vi "MISSION_ITEM Jump.vi"(0 "Waypoint to jump to":sgl, 5 "Number of times to repeat":sgl) -> (4 "Mission Item":T1={"target_system"=0, "target_component"=0, "sequence"=0, "frame"=enum."GLOBAL RELATIVE ALT", "command"=0, "current"=FALSE, "autocontinue"=FALSE, "param1"=0.0, "param2"=0.0, "param3"=0.0, "param4"=0.0, "Lat"=0.0, "Lon"=0.0, "Altitude (m)"=0.0})   [LabVIEW 2014]
uses:
  Controls/Mission Planning Controls/MAVLINK Mission Item.ctl
  Controls/MAVLINK Mav Frame.ctl
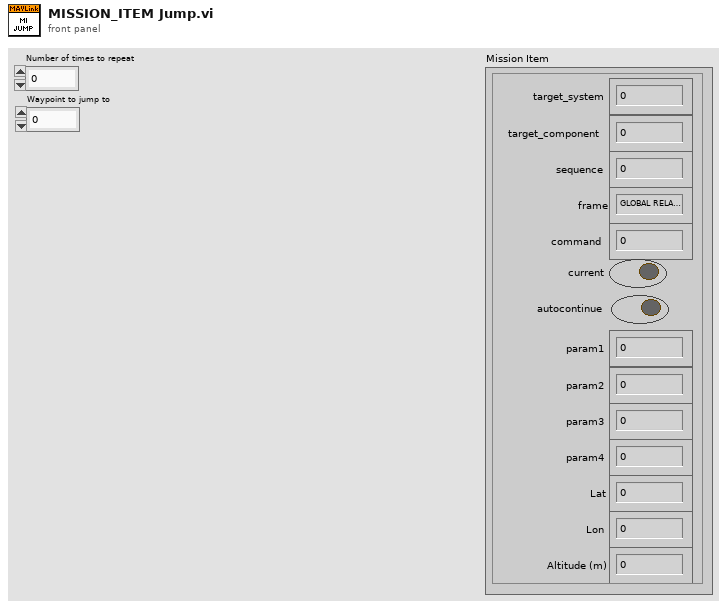
[diagram p1: front panel]
types:
  T1 = typedef "MAVLINK Mission Item.ctl" = cluster{"target_system":u8, "target_component":u8, "sequence":u16, "frame":T2, "command":u16, "current":bool, "autocontinue":bool, "param1":sgl, "param2":sgl, "param3":sgl, "param4":sgl, "Lat":sgl, "Lon":sgl, "Altitude (m)":sgl}
  T2 = typedef "MAVLINK Mav Frame.ctl" = enum8{"GLOBAL", "LOCAL NED", "MISSION", "GLOBAL RELATIVE ALT", "LOCAL ENU", "GLOBAL INT", "GLOBAL RELATIVE ALT INT", "LOCAL OFFSET NED", "BODY NED", "BODY OFFSET NED", "GLOBAL TERRAIN ALT", "GLOBAL TERRAIN ALT INT"}
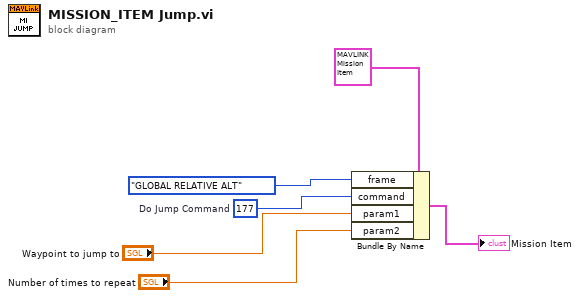
[diagram p0: block diagram]
diagram:
  w6 = u16 177  # Do Jump Command
  n1 = Bundle By Name(cluster=T1 {"target_system"=0, "target_component"=0, "sequence"=0, "frame"=enum."GLOBAL RELATIVE ALT", "command"=0, "current"=FALSE, "autocontinue"=FALSE, "param1"=0.0, "param2"=0.0, "param3"=0.0, "param4"=0.0, "Lat"=0.0, "Lon"=0.0, "Altitude (m)"=0.0} ("MISSION_ITEM"), "frame"=MAVLINK_Mav_Frame."GLOBAL RELATIVE ALT", "command"=w6, "param1"="Waypoint to jump to", "param2"="Number of times to repeat") -> (→"Mission Item":T1)
